vi "WT_main.vi"() -> ()   [LabVIEW 2011]
uses:
  <vilib>/picture/picture.llb/Draw True-Color Pixmap.vi
  <vilib>/imath/engines/lvmath2/RunTimeEngine/ErrorHandling/NIMS_Finalize Error.vi
  <vilib>/imath/engines/lvmath2/RunTimeEngine/VariableToken/NIMS_VariableToken_CondDefined.vi
  <instcachedir>/0/NIMS_VariableToken_CondDefined_D0ABB56CED563FDB50C6D870511BC13F.lvgen/NIMS_VariableToken_CondDefined_D0ABB56CED563FDB50C6D870511BC13F_001.vi
  <vilib>/imathl/engines/lvmath/Functions/Error Handling/Create Error.vi
  <vilib>/imath/engines/lvmath/Functions/Error Handling/MergeErrorsWrapper.vi
  <vilib>/imath/engines/lvmath2/RunTimeEngine/NodeEndStatement/NIMS_NodeEndStatement_Output.vi
  <instcachedir>/0/NIMS_NodeEndStatement_Output_53EC0D466D134D7ABD903AC30B43404B.lvgen/NIMS_NodeEndStatement_Output_53EC0D466D134D7ABD903AC30B43404B_001.vi
  <instcachedir>/0/NIMS_NodeEndStatement_Output_53EC0D466D134D7ABD903AC30B43404B.lvgen/NIMS_NodeEndStatement_Output_53EC0D466D134D7ABD903AC30B43404B_002.vi
  home/anser/natinst/LabVIEW Data/MathScriptVIs/MCStatic_285220864_0ad1dbc67dbced3e2666e8c0598e3af7.vi
  <instcachedir>/0/MCStatic_285220864_0ad1dbc67dbced3e2666e8c0598e3af7_A5E7BD3C14163FD202497231AB81E73F.lvgen/MCStatic_285220864_0ad1dbc67dbced3e2666e8c0598e3af7_A5E7BD3C14163FD202497231AB81E73F_000.vi
  <vilib>/imath/engines/lvmath2/RunTimeEngine/UserFunctionToken/NIMS_UserFunction_CondDefined.vi
  <instcachedir>/0/NIMS_UserFunction_CondDefined_DEFBE50AECD73FE86202036B35C4EF3F.lvgen/NIMS_UserFunction_CondDefined_DEFBE50AECD73FE86202036B35C4EF3F_000.vi
  home/anser/natinst/LabVIEW Data/controller.m
panel:
  out "Waveform Chart 4":dynamicdata(graph)
  out "Waveform Chart 3":dynamicdata(graph)
  out "Waveform Chart 2":dynamicdata(graph)
  out "Waveform Chart":dynamicdata(graph)
  out "BSN":u8
  out "lock":u8
  in  "Path for log file":path
  out "GTS Sensor":T1
  out "Apparatus F":T2 {"volt1" format="%.2f"; "A.2" format="%.2f"; "Tank 2" scale=0.0..20.0; "A.1" format="%.2f"; "Tank 1" scale=0.0..20.0}
  out "Apparatus E":T2 {"volt1" format="%.2f"; "A.2" format="%.2f"; "Tank 2" scale=0.0..20.0; "A.1" format="%.2f"; "Tank 1" scale=0.0..20.0}
  out "Apparatus D":T2 {"volt1" format="%.2f"; "A.2" format="%.2f"; "Tank 2" scale=0.0..20.0; "A.1" format="%.2f"; "Tank 1" scale=0.0..20.0}
  out "Apparatus C":T2 {"volt1" format="%.2f"; "A.2" format="%.2f"; "Tank 2" scale=0.0..20.0; "A.1" format="%.2f"; "Tank 1" scale=0.0..20.0}
  out "ApparatusB":T2 {"volt1" format="%.2f"; "A.2" format="%.2f"; "Tank 2" scale=0.0..20.0; "Tank 1" scale=0.0..20.0}
  out "Apparatus A":T2 {"volt1" format="%.2f"; "A.2" format="%.2f"; "Tank 2" scale=0.0..20.0; "A.1" format="%.2f"; "Tank 1" scale=0.0..20.0}
  in  "Maximum Water Level":dbl=15.0 min=5.0 max=20.0
  in  "Test":dbl=63.0 min=0.0 max=63.0 step=1.0
  out "Actuator_GTS":u8 max=1
  out "Sensor_GTS":u8 max=1
  in  "Controller Mode":dbl=1.0 min=1.0 max=2.0
  in  "Referece Value":dbl=5.0 min=0.0 max=10.0
  out "Packet Sent":string
  out "Packet Received":string
  in  "write":i32=9002
  out "KTH  Automatic Control \nTemplates. Water Tank Project (GTS)\nSerialForwarder-Mote":picture
  in  "Read":i32=9002
  in  "enabled":bool
  # "For Debugging purpose"
  # "Controller Peramerters"
  # "Network Cooridinated Serial Port"
  # "Actuator Id"
  # "Actuator Id"
  # "Actuator Id"
  # "Actuator Id"
  # "Actuator Id"
  # "Actuator Id"
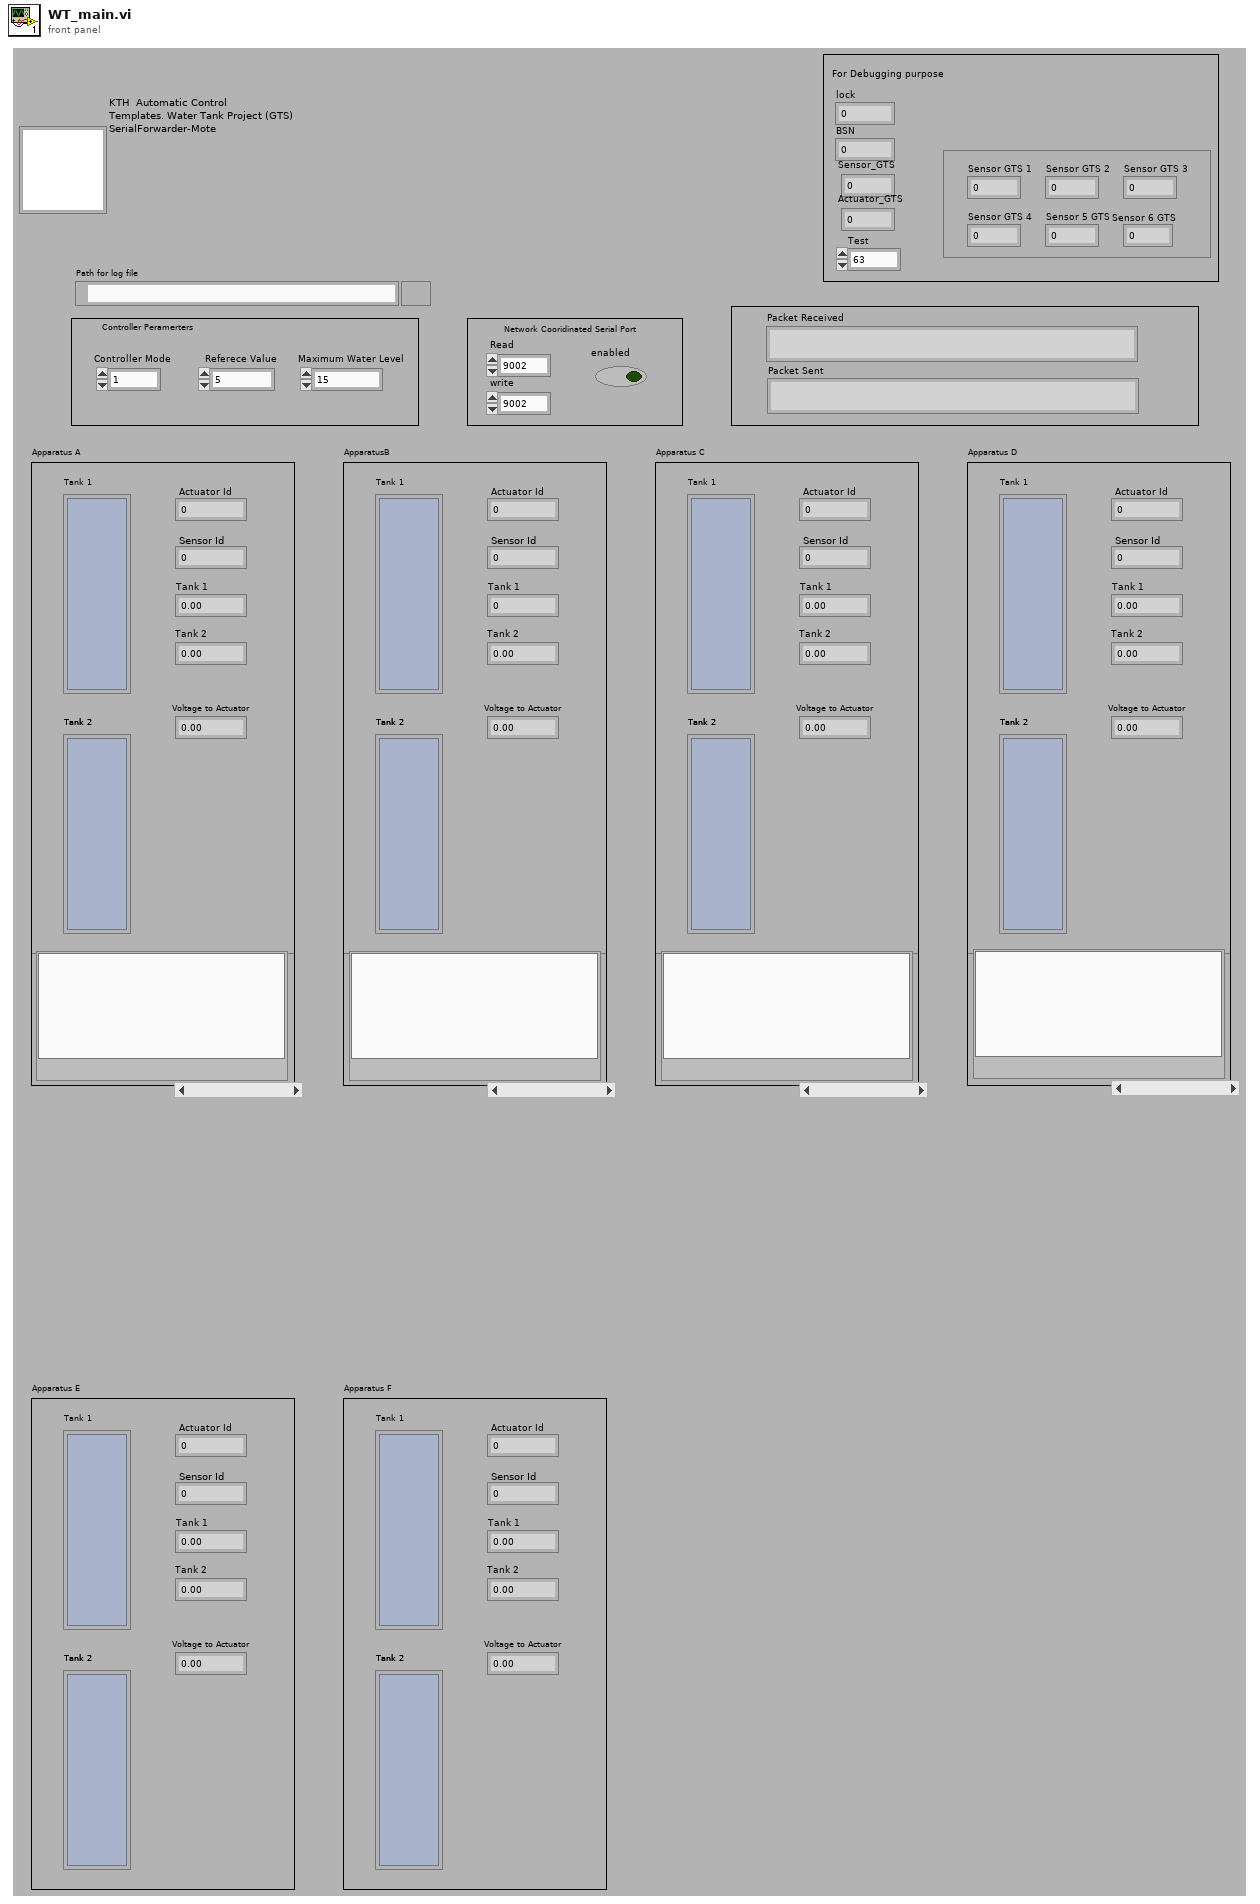
[diagram p1: front panel]
types:
  T1 = cluster{"Sensor 6 GTS":u8, "Sensor 5 GTS":u8, "Sensor GTS 4":u8, "Sensor GTS 3":u8, "Sensor GTS 2":u8, "Sensor GTS 1":u8}
  T2 = cluster{"Tank 1":dbl, "A.1":dbl, "Tank 2":dbl, "A.2":dbl, "    Sensor Id 1":dbl, "Actuator Id 1":dbl, "volt1":dbl}
  T3 = enum16{"open", "replace", "create", "open or create", "replace or create", "replace or create with confirmation"}
  T4 = cluster{dbl, dbl, dbl, dbl, "y":dbl, "sp float":u8}
  T5 = cluster{"Id 6":u8, "ID 5":u8, "Id 4":u8, "Id 3":u8, "Id 2":u8, "Id 1":u8}
  T6 = cluster{dbl, dbl, dbl, dbl, "y":dbl, "sp float":u8, dbl}
  T7 = typedef "imagedata.ctl" = cluster{"image type":i32, "image depth":i32, "image":u8[], "mask":u8[], "colors":u32[], "Rectangle":cluster{"left":i16, "top":i16, "right":i16, "bottom":i16}}
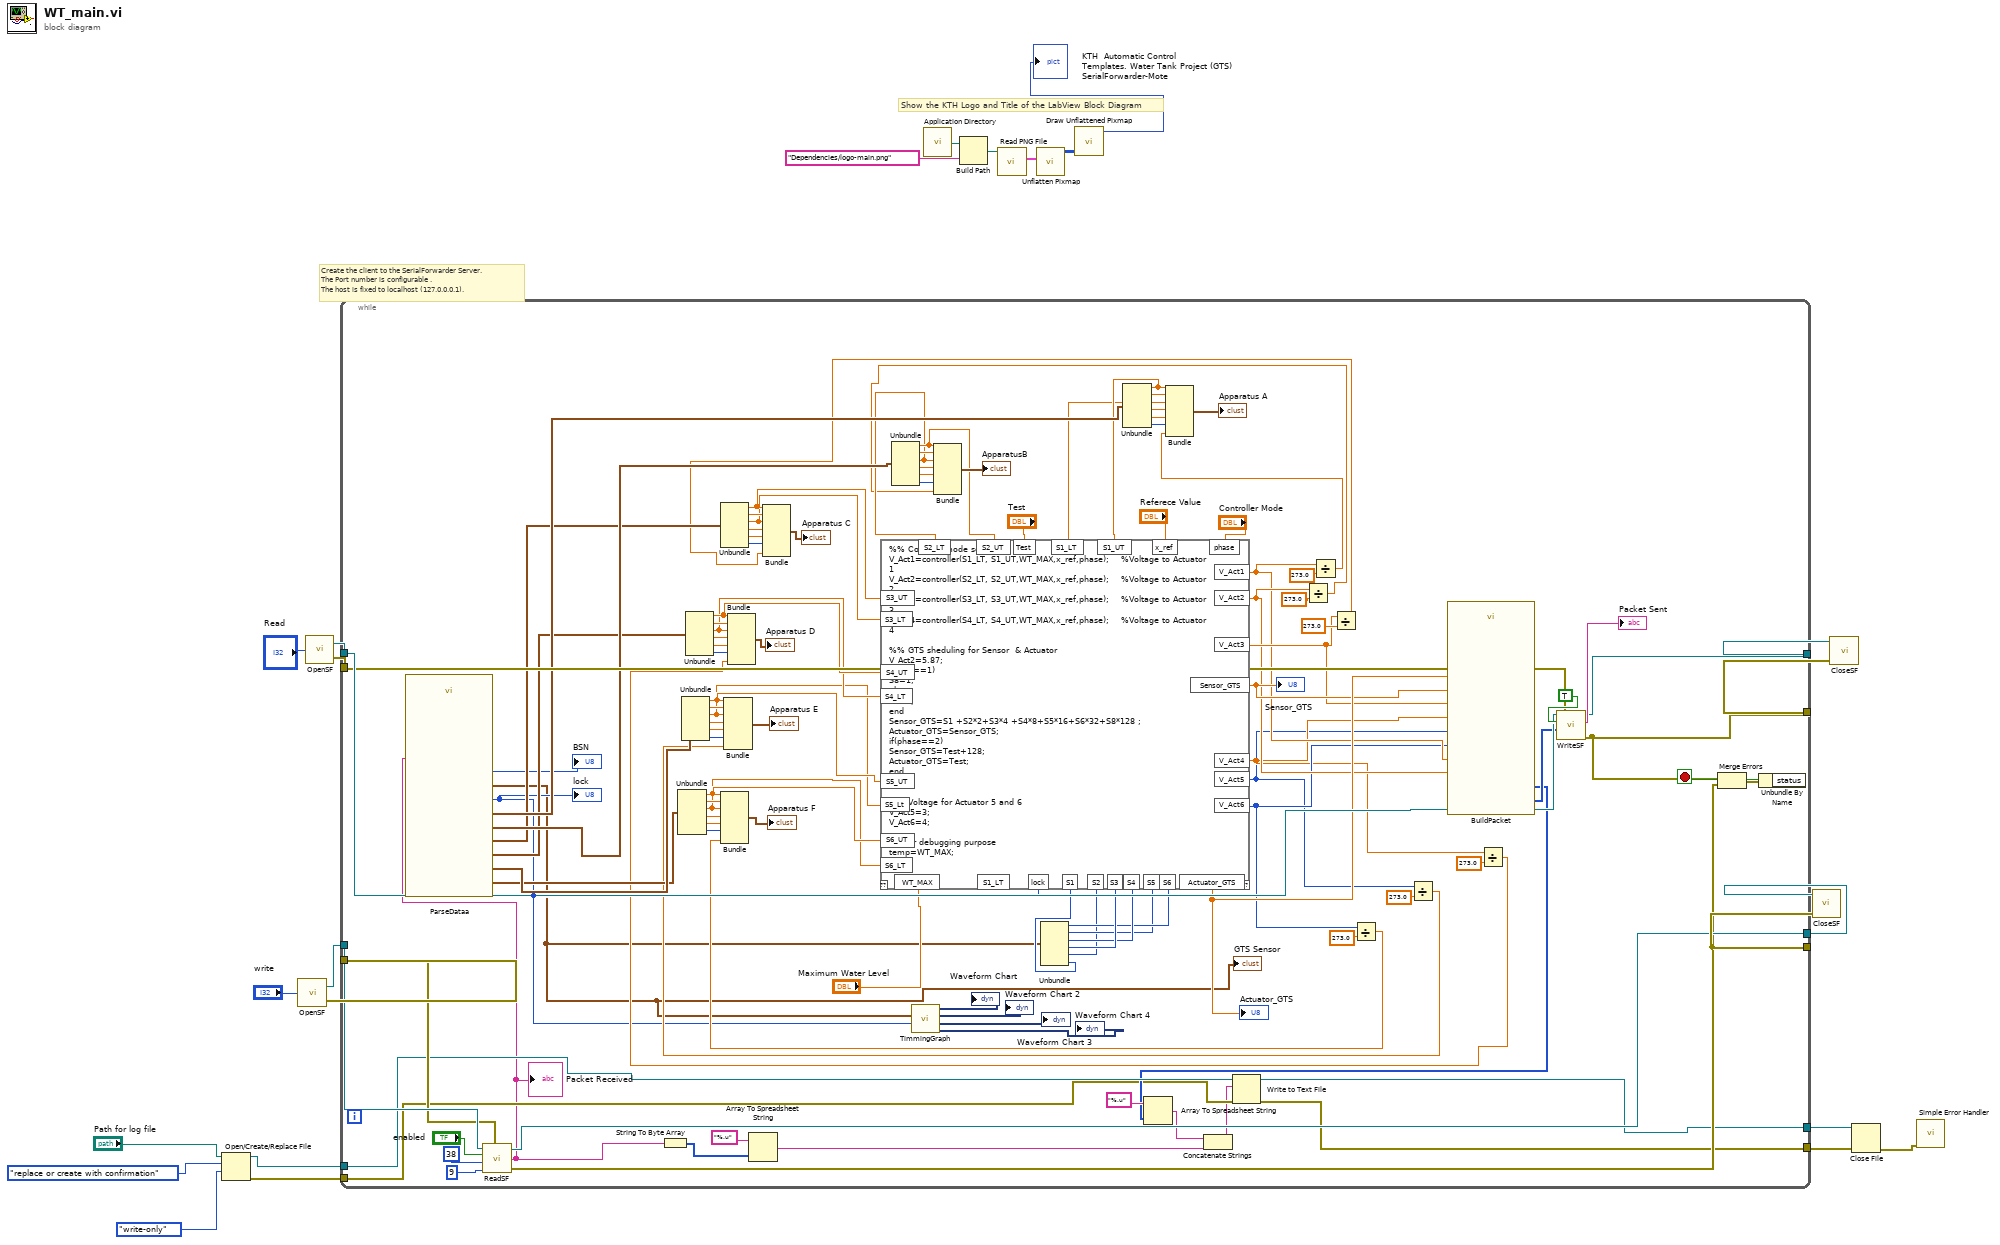
[diagram p0: block diagram]
diagram:
  # "Create the client to the SerialForwarder Server.\nThe Port number is configurable . \nThe host is fixed to localhost (127.0.0.0.1)."
  # "Show the KTH Logo and Title of the LabView Block Diagram"
  n1 = Open/Create/Replace File(file path (use dialog)="Path for log file", operation (0:open)=T3."replace or create with confirmation", access (0:read/write)=enum16{"read/write", "read-only", "write-only"}."write-only") -> (refnum out=w6:refnum<file>, error out=w7:errorcluster)  [unwired: 3 in, 1 out]
  n2 = call "OpenSF.vi"("Port Number"="write") -> ("error out"=w13:errorcluster, "connection ID"=w12:refnum<k5>)
  n3 = call "OpenSF.vi"("Port Number"="Read") -> ("error out"=w18:errorcluster, "connection ID"=w19:refnum<k5>)
  n4 = while {
    tunnel: w19 -> [w128]
    tunnel: w18 -> [w127]
    tunnel: [w130] -> w17
    tunnel: w12 -> [w126]
    tunnel: w13 -> [w125]
    tunnel: [w123] -> w11
    tunnel: [w124] -> w10
    tunnel: [w129] -> w9
    tunnel: w7 -> [w39]
    tunnel: w6 -> [w43]
    tunnel: [w44] -> w5
    tunnel: [w45] -> w4
    stop <- w136 stop-if-true
    n5 = call "ReadSF.vi"("connection ID in"=w126, "error in"=w125, "enabled"="enabled", "bytes to read"=38, "header size"=9) -> ("connection ID out"=w129:refnum<k5>, "string"=w38:string, "error out"=w124:errorcluster)  [unwired: 1 in]
    "Packet Received" <- w38
    n6 = call "ParseDataa.vi"("data out"=w38) -> ("Sensor data 4"=w78:T4, "Sensor data 3"=w84:T4, "Sensor data 2"=w90:T4, "Sensor data 1"=w97:T4, "Sensor data 6"=w66:T4, "Sensor data 5"=w72:T4, "BSN"=→"BSN":u8, "lock"=w30:u8, "GTS Fields"=w28:T5)  [unwired: 2 in]
    "GTS Sensor" <- w28
    "lock" <- w30
    n7 = String To Byte Array(string=w38) -> (unsigned byte array=w37:u8[])
    n8 = Unbundle(w66) -> (w55:dbl, w68:dbl, w54:dbl, w69:dbl, "y"=w70:dbl, "sp float"=w71:u8)
    n9 = Unbundle(w72) -> (w57:dbl, w77:dbl, w56:dbl, w76:dbl, "y"=w75:dbl, "sp float"=w74:u8)
    n10 = Unbundle(w78) -> (w59:dbl, w80:dbl, w58:dbl, w81:dbl, "y"=w82:dbl, "sp float"=w83:u8)
    n11 = Unbundle(w84) -> (w61:dbl, w89:dbl, w60:dbl, w88:dbl, "y"=w87:dbl, "sp float"=w86:u8)
    n12 = Array To Spreadsheet String(array=w37, 3:"%.u") -> (spreadsheet string=w36:string)  [unwired: 1 out]
    n13 = Unbundle(w90) -> (w63:dbl, w92:dbl, w62:dbl, w93:dbl, "y"=w94:dbl, "sp float"=w95:u8)
    n14 = call "TimmingGraph.vi"("lock"=w30, "Cluster"=w28) -> ("Waveform Graph 4"=→"Waveform Chart 4":dynamicdata, "Waveform Graph 3"=→"Waveform Chart 3":dynamicdata, "Waveform Graph 2"=→"Waveform Chart 2":dynamicdata, "Waveform Graph"=→"Waveform Chart":dynamicdata)  [unwired: 6 in]
    n15 = Unbundle(w28) -> ("Id 6"=w115:u8, "ID 5"=w104:u8, "Id 4"=w116:u8, "Id 3"=w117:u8, "Id 2"=w103:u8, "Id 1"=w31:u8)
    n16 = Unbundle(w97) -> (w65:dbl, w101:dbl, w64:dbl, w100:dbl, "y"=w99:dbl, "sp float"=w98:u8)
    n17 = mathscript code="%% Contrller mode selection\nV_Act1=controller(S1_LT, S1_UT,WT_MAX,x_ref,phase);    %Voltage to Actuator 1\nV_Act2=controller(S2_LT, S2_UT,WT_MAX,x_ref,phase);    %Voltage to Actuator 2\nV_Act3=controller(S3_LT, S3_UT,WT_MAX,x_ref,phase);    %Voltage to Actuator 3\nV_Act4=controller(S4_LT, S4_UT,WT_MAX,x_ref,phase);    %Voltage to Actuator 4\n\n%% GTS sheduling for Sensor  & Actuator\nV_Act2=5.87;\nif(lock==1)\nS8=1;\nelse\nS8=0;\nend\nSensor_GTS=S1 +S2*2+S3*4 +S4*8+S5*16+S6*32+S8*128 ;\nActuator_GTS=Sensor_GTS;\nif(phase==2)\nSensor_GTS=Test+128;\nActuator_GTS=Test;\nend\n\n\n%% Voltage for Actuator 5 and 6 \nV_Act5=3;\nV_Act6=4;\n\n%%for debugging purpose\ntemp=WT_MAX;"("S1_LT"=w64, "S1_UT"=w65, "x_ref"="Referece Value", "phase"="Controller Mode", "S2_UT"=w63, "S2_LT"=w62, "S2"=w103, "S3"=w117, "S4"=w116, "S1"=w31, "S5"=w104, "S6"=w115, "S3_UT"=w61, "S3_LT"=w60, "S4_UT"=w59, "S4_LT"=w58, "S5_UT"=w57, "S5_Lt"=w56, "S6_UT"=w55, "S6_LT"=w54, "Test"="Test", "WT_MAX"="Maximum Water Level", "lock"=w30) -> ("V_Act1"=w105:dbl, "V_Act2"=w106:dbl, "Sensor_GTS"=w118:dbl, "Actuator_GTS"=w119:dbl, "V_Act3"=w112:dbl, "V_Act4"=w50:dbl, "V_Act5"=w49:i32, "V_Act6"=w102:i32)  [unwired: 1 in, 2 out]
    "Sensor_GTS" <- w118
    "Actuator_GTS" <- w119
    n18 = Divide(x=w106, y=273.0) -> (x/y=w47:dbl)
    n19 = Bundle(w63, w92, w62, w93, "y"=w94, "sp float"=w95, w47) -> (→"ApparatusB":T6)  [unwired: 1 in]
    n20 = Divide(x=w105, y=273.0) -> (x/y=w48:dbl)
    n21 = Bundle(w65, w101, w64, w100, "y"=w99, "sp float"=w98, w48) -> (→"Apparatus A":T6)  [unwired: 1 in]
    n22 = Divide(x=w112, y=273.0) -> (x/y=w46:dbl)
    n23 = Bundle(w61, w89, w60, w88, "y"=w87, "sp float"=w86, w46) -> (→"Apparatus C":T6)  [unwired: 1 in]
    n24 = Divide(x=w102, y=273.0) -> (x/y=w53:dbl)
    n25 = Bundle(w55, w68, w54, w69, "y"=w70, "sp float"=w71, w53) -> (→"Apparatus F":T6)  [unwired: 1 in]
    n26 = Divide(x=w49, y=273.0) -> (x/y=w52:dbl)
    n27 = Bundle(w57, w77, w56, w76, "y"=w75, "sp float"=w74, w52) -> (→"Apparatus E":T6)  [unwired: 1 in]
    n28 = call "BuildPacket.vi"("Volt 6"=w102, "Volt 5"=w49, "Actuatot GTS"=w119, "Sensor GTS"=w118, "Volt 4"=w50, "Volt2"=w106, "Volt 3"=w112, "Volt1"=w105) -> ("PacketArray"=w41:i32[], "Packet for printing"=w40:i32[])
    n29 = Array To Spreadsheet String(array=w40, 3:"%.u") -> (spreadsheet string=w35:string)  [unwired: 1 out]
    n30 = Concatenate Strings(w35, w36) -> (w34:string)
    n31 = Write to Text File(file (use dialog)=w43, text=w34, error in=w39) -> (refnum out=w44:refnum<file>, error out=w45:errorcluster)  [unwired: 1 in, 1 out]
    n32 = Divide(x=w50, y=273.0) -> (x/y=w51:dbl)
    n33 = Bundle(w59, w80, w58, w81, "y"=w82, "sp float"=w83, w51) -> (→"Apparatus D":T6)  [unwired: 1 in]
    n34 = call "WriteSF.vi"("error in"=w127, "packet"=w41, "Enablle write"=TRUE, "connection ID"=w128) -> ("error out"=w123:errorcluster, "Packet String"=→"Packet Sent":string, "connection ID out"=w130:refnum<k5>)  [unwired: 1 out]
    n35 = Merge Errors(w123, w124) -> (w137:errorcluster)
    n36 = Unbundle By Name(w137) -> ("status"=w136:bool)
  }
  n37 = call <vilib>:"Application Directory.vi"() -> ("Application Directory"=w21:path)
  n38 = Build Path(base path=w21, name or relative path="Dependencies/logo-main.png") -> (appended path=w22:path)
  n39 = call <vilib>:"Read PNG File.vi"("path to PNG file"=w22) -> ("image data"=w24:T7)  [unwired: 8 in, 2 out]
  n40 = call <vilib>:"Unflatten Pixmap.vi"("image data"=w24) -> ("24-bit pixmap"=w23:u32[][])  [unwired: 4 in, 6 out]
  n41 = call-poly <vilib>:"Draw Unflattened Pixmap.vi"("data (RGB format)"=w23) -> ("new picture"=→"KTH  Automatic Control \nTemplates. Water Tank Project (GTS)\nSerialForwarder-Mote":picture)  [unwired: 8 in]
  n42 = call "CloseSF.vi"("error out"=w10, "connection ID"=w9) -> ()  [unwired: 1 in]
  n43 = call "CloseSF.vi"("error out"=w11, "connection ID"=w17) -> ()  [unwired: 1 in]
  n44 = Close File(refnum=w5, error in=w4) -> (error out=w2:errorcluster)  [unwired: 1 out]
  n45 = call <vilib>:"Simple Error Handler.vi"("error in (no error)"=w2) -> ()  [unwired: 1 in, 8 out]
